vi "test TCX read (installed 71).vi"() -> ()   [LabVIEW 2011] (continued)
T14:01:31Z</Time><Position><LatitudeDegrees>35.863725</LatitudeDegrees><LongitudeDegrees>-78.910687</LongitudeDegrees></Position><AltitudeMeters>93.385</AltitudeMeters><DistanceMeters>7071.063</DistanceMeters><Cadence>74</Cadence><Extensions><TPX xmlns=\"http://www.garmin.com/xmlschemas/ActivityExtension/v2\"><Watts>109</Watts></TPX></Extensions></Trackpoint><Trackpoint><Time>2008-03-03T14:01:32Z</Time><Position><LatitudeDegrees>35.863710</LatitudeDegrees><LongitudeDegrees>-78.910596</LongitudeDegrees></Position><AltitudeMeters>93.385</AltitudeMeters><DistanceMeters>7079.492</DistanceMeters><Cadence>74</Cadence><Extensions><TPX xmlns=\"http://www.garmin.com/xmlschemas/ActivityExtension/v2\"><Watts>108</Watts></TPX></Extensions></Trackpoint><Trackpoint><Time>2008-03-03T14:01:33Z</Time><Position><LatitudeDegrees>35.863695</LatitudeDegrees><LongitudeDegrees>-78.910502</LongitudeDegrees></Position><AltitudeMeters>92.905</AltitudeMeters><DistanceMeters>7088.167</DistanceMeters><Cadence>70</Cadence><Extensions><TPX xmlns=\"http://www.garmin.com/xmlschemas/ActivityExtension/v2\"><Watts>110</Watts></TPX></Extensions></Trackpoint><Trackpoint><Time>2008-03-03T14:01:34Z</Time><Position><LatitudeDegrees>35.863685</LatitudeDegrees><LongitudeDegrees>-78.910407</LongitudeDegrees></Position><AltitudeMeters>92.905</AltitudeMeters><DistanceMeters>7096.799</DistanceMeters><Cadence>71</Cadence><Extensions><TPX xmlns=\"http://www.garmin.com/xmlschemas/ActivityExtension/v2\"><Watts>119</Watts></TPX></Extensions></Trackpoint><Trackpoint><Time>2008-03-03T14:01:35Z</Time><Position><LatitudeDegrees>35.863670</LatitudeDegrees><LongitudeDegrees>-78.910309</LongitudeDegrees></Position><AltitudeMeters>92.424</AltitudeMeters><DistanceMeters>7105.804</DistanceMeters><Cadence>74</Cadence><Extensions><TPX xmlns=\"http://www.garmin.com/xmlschemas/ActivityExtension/v2\"><Watts>107</Watts></TPX></Extensions></Trackpoint><Trackpoint><Time>2008-03-03T14:01:36Z</Time><Position><LatitudeDegrees>35.863654</LatitudeDegrees><LongitudeDegrees>-78.910210</LongitudeDegrees></Position><AltitudeMeters>92.424</AltitudeMeters><DistanceMeters>7114.917</DistanceMeters><Cadence>75</Cadence><Extensions><TPX xmlns=\"http://www.garmin.com/xmlschemas/ActivityExtension/v2\"><Watts>96</Watts></TPX></Extensions></Trackpoint><Trackpoint><Time>2008-03-03T14:01:37Z</Time><Position><LatitudeDegrees>35.863638</LatitudeDegrees><LongitudeDegrees>-78.910109</LongitudeDegrees></Position><AltitudeMeters>91.463</AltitudeMeters><DistanceMeters>7124.211</DistanceMeters><Cadence>76</Cadence><Extensions><TPX xmlns=\"http://www.garmin.com/xmlschemas/ActivityExtension/v2\"><Watts>95</Watts></TPX></Extensions></Trackpoint><Trackpoint><Time>2008-03-03T14:01:38Z</Time><Position><LatitudeDegrees>35.863622</LatitudeDegrees><LongitudeDegrees>-78.910006</LongitudeDegrees></Position><AltitudeMeters>91.463</AltitudeMeters><DistanceMeters>7133.708</DistanceMeters><Cadence>77</Cadence><Extensions><TPX xmlns=\"http://www.garmin.com/xmlschemas/ActivityExtension/v2\"><Watts>98</Watts></TPX></Extensions></Trackpoint><Trackpoint><Time>2008-03-03T14:01:39Z</Time><Position><LatitudeDegrees>35.863607</LatitudeDegrees><LongitudeDegrees>-78.909902</LongitudeDegrees></Position><AltitudeMeters>90.982</AltitudeMeters><DistanceMeters>7143.275</DistanceMeters><Cadence>77</Cadence><Extensions><TPX xmlns=\"http://www.garmin.com/xmlschemas/ActivityExtension/v2\"><Watts>98</Watts></TPX></Extensions></Trackpoint><Trackpoint><Time>2008-03-03T14:01:40Z</Time><Position><LatitudeDegrees>35.863592</LatitudeDegrees><LongitudeDegrees>-78.909796</LongitudeDegrees></Position><AltitudeMeters>90.982</AltitudeMeters><DistanceMeters>7152.969</DistanceMeters><Cadence>79</Cadence><Extensions><TPX xmlns=\"http://www.garmin.com/xmlschemas/ActivityExtension/v2\"><Watts>114</Watts></TPX></Extensions></Trackpoint><Trackpoint><Time>2008-03-03T14:01:41Z</Time><Position><LatitudeDegrees>35.863576</LatitudeDegrees><LongitudeDegrees>-78.909689</LongitudeDegrees></Position><AltitudeMeters>90.982</AltitudeMeters><DistanceMeters>7162.816</DistanceMeters><Cadence>80</Cadence><Extensions><TPX xmlns=\"http://www.garmin.com/xmlschemas/ActivityExtension/v2\"><Watts>119</Watts></TPX></Extensions></Trackpoint><Trackpoint><Time>2008-03-03T14:01:42Z</Time><Position><LatitudeDegrees>35.863561</LatitudeDegrees><LongitudeDegrees>-78.909581</LongitudeDegrees></Position><AltitudeMeters>90.982</AltitudeMeters><DistanceMeters>7172.724</DistanceMeters><Cadence>81</Cadence><Extensions><TPX xmlns=\"http://www.garmin.com/xmlschemas/ActivityExtension/v2\"><Watts>127</Watts></TPX></Extensions></Trackpoint><Trackpoint><Time>2008-03-03T14:01:43Z</Time><Position><LatitudeDegrees>35.863542</LatitudeDegrees><LongitudeDegrees>-78.909472</LongitudeDegrees></Position><AltitudeMeters>90.501</AltitudeMeters><DistanceMeters>7182.813</DistanceMeters><Cadence>82</Cadence><Extensions><TPX xmlns=\"http://www.garmin.com/xmlschemas/ActivityExtension/v2\"><Watts>113</Watts></TPX></Extensions></Trackpoint><Trackpoint><Time>2008-03-03T14:01:44Z</Time><Position><LatitudeDegrees>35.863526</LatitudeDegrees><LongitudeDegrees>-78.909363</LongitudeDegrees></Position><AltitudeMeters>90.021</AltitudeMeters><DistanceMeters>7192.831</DistanceMeters><Cadence>82</Cadence><Extensions><TPX xmlns=\"http://www.garmin.com/xmlschemas/ActivityExtension/v2\"><Watts>120</Watts></TPX></Extensions></Trackpoint><Trackpoint><Time>2008-03-03T14:01:45Z</Time><Position><LatitudeDegrees>35.863510</LatitudeDegrees><LongitudeDegrees>-78.909253</LongitudeDegrees></Position><AltitudeMeters>89.540</AltitudeMeters><DistanceMeters>7202.898</DistanceMeters><Cadence>82</Cadence><Extensions><TPX xmlns=\"http://www.garmin.com/xmlschemas/ActivityExtension/v2\"><Watts>110</Watts></TPX></Extensions></Trackpoint><Trackpoint><Time>2008-03-03T14:01:46Z</Time><Position><LatitudeDegrees>35.863491</LatitudeDegrees><LongitudeDegrees>-78.909143</LongitudeDegrees></Position><AltitudeMeters>89.540</AltitudeMeters><DistanceMeters>7213.067</DistanceMeters><Cadence>83</Cadence><Extensions><TPX xmlns=\"http://www.garmin.com/xmlschemas/ActivityExtension/v2\"><Watts>105</Watts></TPX></Extensions></Trackpoint><Trackpoint><Time>2008-03-03T14:01:47Z</Time><Position><LatitudeDegrees>35.863470</LatitudeDegrees><LongitudeDegrees>-78.909031</LongitudeDegrees></Position><AltitudeMeters>89.540</AltitudeMeters><DistanceMeters>7223.420</DistanceMeters><Cadence>83</Cadence><Extensions><TPX xmlns=\"http://www.garmin.com/xmlschemas/ActivityExtension/v2\"><Watts>109</Watts></TPX></Extensions></Trackpoint><Trackpoint><Time>2008-03-03T14:01:48Z</Time><Position><LatitudeDegrees>35.863450</LatitudeDegrees><LongitudeDegrees>-78.908921</LongitudeDegrees></Position><AltitudeMeters>89.059</AltitudeMeters><DistanceMeters>7233.568</DistanceMeters><Cadence>83</Cadence><Extensions><TPX xmlns=\"http://www.garmin.com/xmlschemas/ActivityExtension/v2\"><Watts>110</Watts></TPX></Extensions></Trackpoint><Trackpoint><Time>2008-03-03T14:01:49Z</Time><Position><LatitudeDegrees>35.863429</LatitudeDegrees><LongitudeDegrees>-78.908812</LongitudeDegrees></Position><AltitudeMeters>89.059</AltitudeMeters><DistanceMeters>7243.720</DistanceMeters><Cadence>83</Cadence><Extensions><TPX xmlns=\"http://www.garmin.com/xmlschemas/ActivityExtension/v2\"><Watts>111</Watts></TPX></Extensions></Trackpoint><Trackpoint><Time>2008-03-03T14:01:50Z</Time><Position><LatitudeDegrees>35.863409</LatitudeDegrees><LongitudeDegrees>-78.908702</LongitudeDegrees></Position><AltitudeMeters>89.059</AltitudeMeters><DistanceMeters>7253.881</DistanceMeters><Cadence>82</Cadence><Extensions><TPX xmlns=\"http://www.garmin.com/xmlschemas/ActivityExtension/v2\"><Watts>118</Watts></TPX></Extensions></Trackpoint><Trackpoint><Time>2008-03-03T14:01:51Z</Time><Position><LatitudeDegrees>35.863386</LatitudeDegrees><LongitudeDegrees>-78.908594</LongitudeDegrees></Position><AltitudeMeters>89.540</AltitudeMeters><DistanceMeters>7263.956</DistanceMeters><Cadence>82</Cadence><Extensions><TPX xmlns=\"http://www.garmin.com/xmlschemas/ActivityExtension/v2\"><Watts>118</Watts></TPX></Extensions></Trackpoint><Trackpoint><Time>2008-03-03T14:01:52Z</Time><Position><LatitudeDegrees>35.863365</LatitudeDegrees><LongitudeDegrees>-78.908487</LongitudeDegrees></Position><AltitudeMeters>89.059</AltitudeMeters><DistanceMeters>7273.903</DistanceMeters><Cadence>80</Cadence><Extensions><TPX xmlns=\"http://www.garmin.com/xmlschemas/ActivityExtension/v2\"><Watts>119</Watts></TPX></Extensions></Trackpoint><Trackpoint><Time>2008-03-03T14:01:53Z</Time><Position><LatitudeDegrees>35.863341</LatitudeDegrees><LongitudeDegrees>-78.908381</LongitudeDegrees></Position><AltitudeMeters>89.059</AltitudeMeters><DistanceMeters>7283.836</DistanceMeters><Cadence>80</Cadence><Extensions><TPX xmlns=\"http://www.garmin.com/xmlschemas/ActivityExtension/v2\"><Watts>124</Watts></TPX></Extensions></Trackpoint><Trackpoint><Time>2008-03-03T14:01:54Z</Time><Position><LatitudeDegrees>35.863310</LatitudeDegrees><LongitudeDegrees>-78.908278</LongitudeDegrees></Position><AltitudeMeters>89.059</AltitudeMeters><DistanceMeters>7293.733</DistanceMeters><Cadence>80</Cadence><Extensions><TPX xmlns=\"http://www.garmin.com/xmlschemas/ActivityExtension/v2\"><Watts>127</Watts></TPX></Extensions></Trackpoint><Trackpoint><Time>2008-03-03T14:01:55Z</Time><Position><LatitudeDegrees>35.863282</LatitudeDegrees><LongitudeDegrees>-78.908177</LongitudeDegrees></Position><AltitudeMeters>88.579</AltitudeMeters><DistanceMeters>7303.308</DistanceMeters><Cadence>77</Cadence><Extensions><TPX xmlns=\"http://www.garmin.com/xmlschemas/ActivityExtension/v2\"><Watts>143</Watts></TPX></Extensions></Trackpoint><Trackpoint><Time>2008-03-03T14:01:56Z</Time><Position><LatitudeDegrees>35.863254</LatitudeDegrees><LongitudeDegrees>-78.908080</LongitudeDegrees></Position><AltitudeMeters>89.059</AltitudeMeters><DistanceMeters>7312.629</DistanceMeters><Cadence>76</Cadence><Extensions><TPX xmlns=\"http://www.garmin.com/xmlschemas/ActivityExtension/v2\"><Watts>158</Watts></TPX></Extensions></Trackpoint><Trackpoint><Time>2008-03-03T14:01:57Z</Time><Position><LatitudeDegrees>35.863228</LatitudeDegrees><LongitudeDegrees>-78.907986</LongitudeDegrees></Position><AltitudeMeters>89.540</AltitudeMeters><DistanceMeters>7321.532</DistanceMeters><Cadence>73</Cadence><Extensions><TPX xmlns=\"http://www.garmin.com/xmlschemas/ActivityExtension/v2\"><Watts>164</Watts></TPX></Extensions></Trackpoint><Trackpoint><Time>2008-03-03T14:01:58Z</Time><Position><LatitudeDegrees>35.863199</LatitudeDegrees><LongitudeDegrees>-78.907895</LongitudeDegrees></Position><AltitudeMeters>89.540</AltitudeMeters><DistanceMeters>7330.394</DistanceMeters><Cadence>70</Cadence><Extensions><TPX xmlns=\"http://www.garmin.com/xmlschemas/ActivityExtension/v2\"><Watts>168</Watts></TPX></Extensions></Trackpoint><Trackpoint><Time>2008-03-03T14:01:59Z</Time><Position><LatitudeDegrees>35.863176</LatitudeDegrees><LongitudeDegrees>-78.907807</LongitudeDegrees></Position><AltitudeMeters>89.540</AltitudeMeters><DistanceMeters>7338.662</DistanceMeters><Cadence>70</Cadence><Extensions><TPX xmlns=\"http://www.garmin.com/xmlschemas/ActivityExtension/v2\"><Watts>170</Watts></TPX></Extensions></Trackpoint><Trackpoint><Time>2008-03-03T14:02:00Z</Time><Position><LatitudeDegrees>35.863156</LatitudeDegrees><LongitudeDegrees>-78.907723</LongitudeDegrees></Position><AltitudeMeters>89.540</AltitudeMeters><DistanceMeters>7346.539</DistanceMeters><Cadence>76</Cadence><Extensions><TPX xmlns=\"http://www.garmin.com/xmlschemas/ActivityExtension/v2\"><Watts>163</Watts></TPX></Extensions></Trackpoint><Trackpoint><Time>2008-03-03T14:02:01Z</Time><Position><LatitudeDegrees>35.863135</LatitudeDegrees><LongitudeDegrees>-78.907643</LongitudeDegrees></Position><AltitudeMeters>89.540</AltitudeMeters><DistanceMeters>7354.126</DistanceMeters><Cadence>80</Cadence><Extensions><TPX xmlns=\"http://www.garmin.com/xmlschemas/ActivityExtension/v2\"><Watts>164</Watts></TPX></Extensions></Trackpoint><Trackpoint><Time>2008-03-03T14:02:02Z</Time><Position><LatitudeDegrees>35.863115</LatitudeDegrees><LongitudeDegrees>-78.907565</LongitudeDegrees></Position><AltitudeMeters>90.501</AltitudeMeters><DistanceMeters>7361.460</DistanceMeters><Cadence>77</Cadence><Extensions><TPX xmlns=\"http://www.garmin.com/xmlschemas/ActivityExtension/v2\"><Watts>190</Watts></TPX></Extensions></Trackpoint><Trackpoint><Time>2008-03-03T14:02:03Z</Time><Position><LatitudeDegrees>35.863091</LatitudeDegrees><LongitudeDegrees>-78.907489</LongitudeDegrees></Position><AltitudeMeters>90.501</AltitudeMeters><DistanceMeters>7368.861</DistanceMeters><Cadence>76</Cadence><Extensions><TPX xmlns=\"http://www.garmin.com/xmlschemas/ActivityExtension/v2\"><Watts>233</Watts></TPX></Extensions></Trackpoint><Trackpoint><Time>2008-03-03T14:02:04Z</Time><Position><LatitudeDegrees>35.863071</LatitudeDegrees><LongitudeDegrees>-78.907413</LongitudeDegrees></Position><AltitudeMeters>90.501</AltitudeMeters><DistanceMeters>7376.071</DistanceMeters><Cadence>76</Cadence><Extensions><TPX xmlns=\"http://www.garmin.com/xmlschemas/ActivityExtension/v2\"><Watts>311</Watts></TPX></Extensions></Trackpoint><Trackpoint><Time>2008-03-03T14:02:05Z</Time><Position><LatitudeDegrees>35.863051</LatitudeDegrees><LongitudeDegrees>-78.907336</LongitudeDegrees></Position><AltitudeMeters>90.982</AltitudeMeters><DistanceMeters>7383.323</DistanceMeters><Cadence>76</Cadence><Extensions><TPX xmlns=\"http://www.garmin.com/xmlschemas/ActivityExtension/v2\"><Watts>376</Watts></TPX></Extensions></Trackpoint><Trackpoint><Time>2008-03-03T14:02:06Z</Time><Position><LatitudeDegrees>35.863031</LatitudeDegrees><LongitudeDegrees>-78.907260</LongitudeDegrees></Position><AltitudeMeters>91.463</AltitudeMeters><DistanceMeters>7390.527</DistanceMeters><Cadence>75</Cadence><Extensions><TPX xmlns=\"http://www.garmin.com/xmlschemas/ActivityExtension/v2\"><Watts>375</Watts></TPX></Extensions></Trackpoint><Trackpoint><Time>2008-03-03T14:02:07Z</Time><Position><LatitudeDegrees>35.863008</LatitudeDegrees><LongitudeDegrees>-78.907185</LongitudeDegrees></Position><AltitudeMeters>91.463</AltitudeMeters><DistanceMeters>7397.769</DistanceMeters><Cadence>75</Cadence><Extensions><TPX xmlns=\"http://www.garmin.com/xmlschemas/ActivityExtension/v2\"><Watts>366</Watts></TPX></Extensions></Trackpoint><Trackpoint><Time>2008-03-03T14:02:08Z</Time><Position><LatitudeDegrees>35.862984</LatitudeDegrees><LongitudeDegrees>-78.907112</LongitudeDegrees></Position><AltitudeMeters>91.943</AltitudeMeters><DistanceMeters>7404.936</DistanceMeters><Cadence>73</Cadence><Extensions><TPX xmlns=\"http://www.garmin.com/xmlschemas/ActivityExtension/v2\"><Watts>326</Watts></TPX></Extensions></Trackpoint><Trackpoint><Time>2008-03-03T14:02:09Z</Time><Position><LatitudeDegrees>35.862961</LatitudeDegrees><LongitudeDegrees>-78.907039</LongitudeDegrees></Position><AltitudeMeters>91.943</AltitudeMeters><DistanceMeters>7411.968</DistanceMeters><Cadence>73</Cadence><Extensions><TPX xmlns=\"http://www.garmin.com/xmlschemas/ActivityExtension/v2\"><Watts>326</Watts></TPX></Extensions></Trackpoint><Trackpoint><Time>2008-03-03T14:02:10Z</Time><Position><LatitudeDegrees>35.862937</LatitudeDegrees><LongitudeDegrees>-78.906968</LongitudeDegrees></Position><AltitudeMeters>91.943</AltitudeMeters><DistanceMeters>7418.891</DistanceMeters><Cadence>72</Cadence><Extensions><TPX xmlns=\"http://www.garmin.com/xmlschemas/ActivityExtension/v2\"><Watts>311</Watts></TPX></Extensions></Trackpoint><Trackpoint><Time>2008-03-03T14:02:11Z</Time><Position><LatitudeDegrees>35.862914</LatitudeDegrees><LongitudeDegrees>-78.906899</LongitudeDegrees></Position><AltitudeMeters>92.424</AltitudeMeters><DistanceMeters>7425.608</DistanceMeters><Cadence>70</Cadence><Extensions><TPX xmlns=\"http://www.garmin.com/xmlschemas/ActivityExtension/v2\"><Watts>296</Watts></TPX></Extensions></Trackpoint><Trackpoint><Time>2008-03-03T14:02:12Z</Time><Position><LatitudeDegrees>35.862890</LatitudeDegrees><LongitudeDegrees>-78.906832</LongitudeDegrees></Position><AltitudeMeters>92.424</AltitudeMeters><DistanceMeters>7432.226</DistanceMeters><Cadence>70</Cadence><Extensions><TPX xmlns=\"http://www.garmin.com/xmlschemas/ActivityExtension/v2\"><Watts>283</Watts></TPX></Extensions></Trackpoint><Trackpoint><Time>2008-03-03T14:02:13Z</Time><Position><LatitudeDegrees>35.862866</LatitudeDegrees><LongitudeDegrees>-78.906766</LongitudeDegrees></Position><AltitudeMeters>92.905</AltitudeMeters><DistanceMeters>7438.779</DistanceMeters><Cadence>69</Cadence><Extensions><TPX xmlns=\"http://www.garmin.com/xmlschemas/ActivityExtension/v2\"><Watts>271</Watts></TPX></Extensions></Trackpoint><Trackpoint><Time>2008-03-03T14:02:14Z</Time><Position><LatitudeDegrees>35.862841</LatitudeDegrees><LongitudeDegrees>-78.906700</LongitudeDegrees></Position><AltitudeMeters>92.905</AltitudeMeters><DistanceMeters>7445.341</DistanceMeters><Cadence>68</Cadence><Extensions><TPX xmlns=\"http://www.garmin.com/xmlschemas/ActivityExtension/v2\"><Watts>265</Watts></TPX></Extensions></Trackpoint><Trackpoint><Time>2008-03-03T14:02:15Z</Time><Position><LatitudeDegrees>35.862814</LatitudeDegrees><LongitudeDegrees>-78.906635</LongitudeDegrees></Position><AltitudeMeters>92.905</AltitudeMeters><DistanceMeters>7451.964</DistanceMeters><Cadence>69</Cadence><Extensions><TPX xmlns=\"http://www.garmin.com/xmlschemas/ActivityExtension/v2\"><Watts>259</Watts></TPX></Extensions></Trackpoint><Trackpoint><Time>2008-03-03T14:02:16Z</Time><Position><LatitudeDegrees>35.862788</LatitudeDegrees><LongitudeDegrees>-78.906569</LongitudeDegrees></Position><AltitudeMeters>92.905</AltitudeMeters><DistanceMeters>7458.573</DistanceMeters><Cadence>69</Cadence><Extensions><TPX xmlns=\"http://www.garmin.com/xmlschemas/ActivityExtension/v2\"><Watts>224</Watts></TPX></Extensions></Trackpoint><Trackpoint><Time>2008-03-03T14:02:17Z</Time><Position><LatitudeDegrees>35.862762</LatitudeDegrees><LongitudeDegrees>-78.906502</LongitudeDegrees></Position><AltitudeMeters>93.385</AltitudeMeters><DistanceMeters>7465.271</DistanceMeters><Cadence>70</Cadence><Extensions><TPX xmlns=\"http://www.garmin.com/xmlschemas/ActivityExtension/v2\"><Watts>183</Watts></TPX></Extensions></Trackpoint><Trackpoint><Time>2008-03-03T14:02:18Z</Time><Position><LatitudeDegrees>35.862733</LatitudeDegrees><LongitudeDegrees>-78.906434</LongitudeDegrees></Position><AltitudeMeters>93.385</AltitudeMeters><DistanceMeters>7472.209</DistanceMeters><Cadence>71</Cadence><Extensions><TPX xmlns=\"http://www.garmin.com/xmlschemas/ActivityExtension/v2\"><Watts>175</Watts></TPX></Extensions></Trackpoint><Trackpoint><Time>2008-03-03T14:02:19Z</Time><Position><LatitudeDegrees>35.862707</LatitudeDegrees><LongitudeDegrees>-78.906364</LongitudeDegrees></Position><AltitudeMeters>93.385</AltitudeMeters><DistanceMeters>7479.178</DistanceMeters><Cadence>74</Cadence><Extensions><TPX xmlns=\"http://www.garmin.com/xmlschemas/ActivityExtension/v2\"><Watts>127</Watts></TPX></Extensions></Trackpoint><Trackpoint><Time>2008-03-03T14:02:20Z</Time><Position><LatitudeDegrees>35.862678</LatitudeDegrees><LongitudeDegrees>-78.906293</LongitudeDegrees></Position><AltitudeMeters>93.385</AltitudeMeters><DistanceMeters>7486.349</DistanceMeters><Cadence>76</Cadence><Extensions><TPX xmlns=\"http://www.garmin.com/xmlschemas/ActivityExtension/v2\"><Watts>106</Watts></TPX></Extensions></Trackpoint><Trackpoint><Time>2008-03-03T14:02:21Z</Time><Position><LatitudeDegrees>35.862649</LatitudeDegrees><LongitudeDegrees>-78.906220</LongitudeDegrees></Position><AltitudeMeters>92.905</AltitudeMeters><DistanceMeters>7493.638</DistanceMeters><Cadence>76</Cadence><Extensions><TPX xmlns=\"http://www.garmin.com/xmlschemas/ActivityExtension/v2\"><Watts>105</Watts></TPX></Extensions></Trackpoint><Trackpoint><Time>2008-03-03T14:02:22Z</Time><Position><LatitudeDegrees>35.862616</LatitudeDegrees><LongitudeDegrees>-78.906145</LongitudeDegrees></Position><AltitudeMeters>92.905</AltitudeMeters><DistanceMeters>7501.450</DistanceMeters><Cadence>74</Cadence><Extensions><TPX xmlns=\"http://www.garmin.com/xmlschemas/ActivityExtension/v2\"><Watts>105</Watts></TPX></Extensions></Trackpoint><Trackpoint><Time>2008-03-03T14:02:23Z</Time><Position><LatitudeDegrees>35.862577</LatitudeDegrees><LongitudeDegrees>-78.906066</LongitudeDegrees></Position><AltitudeMeters>92.905</AltitudeMeters><DistanceMeters>7509.722</DistanceMeters><Cadence>74</Cadence><Extensions><TPX xmlns=\"http://www.garmin.com/xmlschemas/ActivityExtension/v2\"><Watts>107</Watts></TPX></Extensions></Trackpoint><Trackpoint><Time>2008-03-03T14:02:24Z</Time><Position><LatitudeDegrees>35.862538</LatitudeDegrees><LongitudeDegrees>-78.905985</LongitudeDegrees></Position><AltitudeMeters>92.424</AltitudeMeters><DistanceMeters>7518.321</DistanceMeters><Cadence>79</Cadence><Extensions><TPX xmlns=\"http://www.garmin.com/xmlschemas/ActivityExtension/v2\"><Watts>149</Watts></TPX></Extensions></Trackpoint><Trackpoint><Time>2008-03-03T14:02:25Z</Time><Position><LatitudeDegrees>35.862503</LatitudeDegrees><LongitudeDegrees>-78.905901</LongitudeDegrees></Position><AltitudeMeters>92.424</AltitudeMeters><DistanceMeters>7526.838</DistanceMeters><Cadence>81</Cadence><Extensions><TPX xmlns=\"http://www.garmin.com/xmlschemas/ActivityExtension/v2\"><Watts>149</Watts></TPX></Extensions></Trackpoint><Trackpoint><Time>2008-03-03T14:02:26Z</Time><Position><LatitudeDegrees>35.862465</LatitudeDegrees><LongitudeDegrees>-78.905813</LongitudeDegrees></Position><AltitudeMeters>91.943</AltitudeMeters><DistanceMeters>7535.852</DistanceMeters><Cadence>84</Cadence><Extensions><TPX xmlns=\"http://www.garmin.com/xmlschemas/ActivityExtension/v2\"><Watts>152</Watts></TPX></Extensions></Trackpoint><Trackpoint><Time>2008-03-03T14:02:27Z</Time><Position><LatitudeDegrees>35.862426</LatitudeDegrees><LongitudeDegrees>-78.905724</LongitudeDegrees></Position><AltitudeMeters>91.463</AltitudeMeters><DistanceMeters>7544.979</DistanceMeters><Cadence>86</Cadence><Extensions><TPX xmlns=\"http://www.garmin.com/xmlschemas/ActivityExtension/v2\"><Watts>137</Watts></TPX></Extensions></Trackpoint><Trackpoint><Time>2008-03-03T14:02:28Z</Time><Position><LatitudeDegrees>35.862387</LatitudeDegrees><LongitudeDegrees>-78.905633</LongitudeDegrees></Position><AltitudeMeters>92.424</AltitudeMeters><DistanceMeters>7554.277</DistanceMeters><Cadence>86</Cadence><Extensions><TPX xmlns=\"http://www.garmin.com/xmlschemas/ActivityExtension/v2\"><Watts>137</Watts></TPX></Extensions></Trackpoint><Trackpoint><Time>2008-03-03T14:02:29Z</Time><Position><LatitudeDegrees>35.862347</LatitudeDegrees><LongitudeDegrees>-78.905540</LongitudeDegrees></Position><AltitudeMeters>91.463</AltitudeMeters><DistanceMeters>7563.752</DistanceMeters><Cadence>88</Cadence><Extensions><TPX xmlns=\"http://www.garmin.com/xmlschemas/ActivityExtension/v2\"><Watts>137</Watts></TPX></Extensions></Trackpoint><Trackpoint><Time>2008-03-03T14:02:30Z</Time><Position><LatitudeDegrees>35.862308</LatitudeDegrees><LongitudeDegrees>-78.905447</LongitudeDegrees></Position><AltitudeMeters>91.463</AltitudeMeters><DistanceMeters>7573.245</DistanceMeters><Cadence>87</Cadence><Extensions><TPX xmlns=\"http://www.garmin.com/xmlschemas/ActivityExtension/v2\"><Watts>150</Watts></TPX></Extensions></Trackpoint><Trackpoint><Time>2008-03-03T14:02:31Z</Time><Position><LatitudeDegrees>35.862269</LatitudeDegrees><LongitudeDegrees>-78.905354</LongitudeDegrees></Position><AltitudeMeters>91.463</AltitudeMeters><DistanceMeters>7582.627</DistanceMeters><Cadence>87</Cadence><Extensions><TPX xmlns=\"http://www.garmin.com/xmlschemas/ActivityExtension/v2\"><Watts>149</Watts></TPX></Extensions></Trackpoint><Trackpoint><Time>2008-03-03T14:02:32Z</Time><Position><LatitudeDegrees>35.862232</LatitudeDegrees><LongitudeDegrees>-78.905262</LongitudeDegrees></Position><AltitudeMeters>91.463</AltitudeMeters><DistanceMeters>7591.958</DistanceMeters><Cadence>86</Cadence><Extensions><TPX xmlns=\"http://www.garmin.com/xmlschemas/ActivityExtension/v2\"><Watts>167</Watts></TPX></Extensions></Trackpoint><Trackpoint><Time>2008-03-03T14:02:33Z</Time><Position><LatitudeDegrees>35.862199</LatitudeDegrees><LongitudeDegrees>-78.905168</LongitudeDegrees></Position><AltitudeMeters>91.463</AltitudeMeters><DistanceMeters>7601.143</DistanceMeters><Cadence>86</Cadence><Extensions><TPX xmlns=\"http://www.garmin.com/xmlschemas/ActivityExtension/v2\"><Watts>166</Watts></TPX></Extensions></Trackpoint><Trackpoint><Time>2008-03-03T14:02:34Z</Time><Position><LatitudeDegrees>35.862167</LatitudeDegrees><LongitudeDegrees>-78.905075</LongitudeDegrees></Position><AltitudeMeters>91.463</AltitudeMeters><DistanceMeters>7610.301</DistanceMeters><Cadence>85</Cadence><Extensions><TPX xmlns=\"http://www.garmin.com/xmlschemas/ActivityExtension/v2\"><Watts>166</Watts></TPX></Extensions></Trackpoint><Trackpoint><Time>2008-03-03T14:02:35Z</Time><Position><LatitudeDegrees>35.862140</LatitudeDegrees><LongitudeDegrees>-78.904980</LongitudeDegrees></Position><AltitudeMeters>91.463</AltitudeMeters><DistanceMeters>7619.282</DistanceMeters><Cadence>83</Cadence><Extensions><TPX xmlns=\"http://www.garmin.com/xmlschemas/ActivityExtension/v2\"><Watts>162</Watts></TPX></Extensions></Trackpoint><Trackpoint><Time>2008-03-03T14:02:36Z</Time><Position><LatitudeDegrees>35.862123</LatitudeDegrees><LongitudeDegrees>-78.904885</LongitudeDegrees></Position><AltitudeMeters>91.463</AltitudeMeters><DistanceMeters>7628.092</DistanceMeters><Cadence>81</Cadence><Extensions><TPX xmlns=\"http://www.garmin.com/xmlschemas/ActivityExtension/v2\"><Watts>154</Watts></TPX></Extensions></Trackpoint><Trackpoint><Time>2008-03-03T14:02:37Z</Time><Position><LatitudeDegrees>35.862111</LatitudeDegrees><LongitudeDegrees>-78.904789</LongitudeDegrees></Position><AltitudeMeters>91.943</AltitudeMeters><DistanceMeters>7636.858</DistanceMeters><Cadence>81</Cadence><Extensions><TPX xmlns=\"http://www.garmin.com/xmlschemas/ActivityExtension/v2\"><Watts>149</Watts></TPX></Extensions></Trackpoint><Trackpoint><Time>2008-03-03T14:02:38Z</Time><Position><LatitudeDegrees>35.862110</LatitudeDegrees><LongitudeDegrees>-78.904692</LongitudeDegrees></Position><AltitudeMeters>91.463</AltitudeMeters><DistanceMeters>7645.604</DistanceMeters><Cadence>81</Cadence><Extensions><TPX xmlns=\"http://www.garmin.com/xmlschemas/ActivityExtension/v2\"><Watts>143</Watts></TPX></Extensions></Trackpoint><Trackpoint><Time>2008-03-03T14:02:39Z</Time><Position><LatitudeDegrees>35.862115</LatitudeDegrees><LongitudeDegrees>-78.904595</LongitudeDegrees></Position><AltitudeMeters>91.463</AltitudeMeters><DistanceMeters>7654.416</DistanceMeters><Cadence>82</Cadence><Extensions><TPX xmlns=\"http://www.garmin.com/xmlschemas/ActivityExtension/v2\"><Watts>129</Watts></TPX></Extensions></Trackpoint><Trackpoint><Time>2008-03-03T14:02:40Z</Time><Position><LatitudeDegrees>35.862128</LatitudeDegrees><LongitudeDegrees>-78.904496</LongitudeDegrees></Position><AltitudeMeters>90.982</AltitudeMeters><DistanceMeters>7663.441</DistanceMeters><Cadence>82</Cadence><Extensions><TPX xmlns=\"http://www.garmin.com/xmlschemas/ActivityExtension/v2\"><Watts>129</Watts></TPX></Extensions></Trackpoint><Trackpoint><Time>2008-03-03T14:02:41Z</Time><Position><LatitudeDegrees>35.862146</LatitudeDegrees><LongitudeDegrees>-78.904397</LongitudeDegrees></Position><AltitudeMeters>90.982</AltitudeMeters><DistanceMeters>7672.676</DistanceMeters><Cadence>85</Cadence><Extensions><TPX xmlns=\"http://www.garmin.com/xmlschemas/ActivityExtension/v2\"><Watts>119</Watts></TPX></Extensions></Trackpoint><Trackpoint><Time>2008-03-03T14:02:42Z</Time><Position><LatitudeDegrees>35.862170</LatitudeDegrees><LongitudeDegrees>-78.904297</LongitudeDegrees></Position><AltitudeMeters>90.982</AltitudeMeters><DistanceMeters>7682.102</DistanceMeters><Cadence>86</Cadence><Extensions><TPX xmlns=\"http://www.garmin.com/xmlschemas/ActivityExtension/v2\"><Watts>117</Watts></TPX></Extensions></Trackpoint><Trackpoint><Time>2008-03-03T14:02:43Z</Time><Position><LatitudeDegrees>35.862199</LatitudeDegrees><LongitudeDegrees>-78.904198</LongitudeDegrees></Position><AltitudeMeters>90.982</AltitudeMeters><DistanceMeters>7691.604</DistanceMeters><Cadence>86</Cadence><Extensions><TPX xmlns=\"http://www.garmin.com/xmlschemas/ActivityExtension/v2\"><Watts>107</Watts></TPX></Extensions></Trackpoint><Trackpoint><Time>2008-03-03T14:02:44Z</Time><Position><LatitudeDegrees>35.862231</LatitudeDegrees><LongitudeDegrees>-78.904100</LongitudeDegrees></Position><AltitudeMeters>90.501</AltitudeMeters><DistanceMeters>7701.092</DistanceMeters><Cadence>87</Cadence><Extensions><TPX xmlns=\"http://www.garmin.com/xmlschemas/ActivityExtension/v2\"><Watts>115</Watts></TPX></Extensions></Trackpoint><Trackpoint><Time>2008-03-03T14:02:45Z</Time><Position><LatitudeDegrees>35.862262</LatitudeDegrees><LongitudeDegrees>-78.904002</LongitudeDegrees></Position><AltitudeMeters>90.501</AltitudeMeters><DistanceMeters>7710.564</DistanceMeters><Cadence>87</Cadence><Extensions><TPX xmlns=\"http://www.garmin.com/xmlschemas/ActivityExtension/v2\"><Watts>113</Watts></TPX></Extensions></Trackpoint><Trackpoint><Time>2008-03-03T14:02:46Z</Time><Position><LatitudeDegrees>35.862294</LatitudeDegrees><LongitudeDegrees>-78.903905</LongitudeDegrees></Position><AltitudeMeters>90.982</AltitudeMeters><DistanceMeters>7720.042</DistanceMeters><Cadence>87</Cadence><Extensions><TPX xmlns=\"http://www.garmin.com/xmlschemas/ActivityExtension/v2\"><Watts>112</Watts></TPX></Extensions></Trackpoint><Trackpoint><Time>2008-03-03T14:02:47Z</Time><Position><LatitudeDegrees>35.862327</LatitudeDegrees><LongitudeDegrees>-78.903811</LongitudeDegrees></Position><AltitudeMeters>90.982</AltitudeMeters><DistanceMeters>7729.342</DistanceMeters><Cadence>85</Cadence><Extensions><TPX xmlns=\"http://www.garmin.com/xmlschemas/ActivityExtension/v2\"><Watts>114</Watts></TPX></Extensions></Trackpoint><Trackpoint><Time>2008-03-03T14:02:48Z</Time><Position><LatitudeDegrees>35.862359</LatitudeDegrees><LongitudeDegrees>-78.903717</LongitudeDegrees></Position><AltitudeMeters>90.501</AltitudeMeters><DistanceMeters>7738.435</DistanceMeters><Cadence>84</Cadence><Extensions><TPX xmlns=\"http://www.garmin.com/xmlschemas/ActivityExtension/v2\"><Watts>114</Watts></TPX></Extensions></Trackpoint><Trackpoint><Time>2008-03-03T14:02:49Z</Time><Position><LatitudeDegrees>35.862388</LatitudeDegrees><LongitudeDegrees>-78.903627</LongitudeDegrees></Position><AltitudeMeters>90.501</AltitudeMeters><DistanceMeters>7747.194</DistanceMeters><Cadence>79</Cadence><Extensions><TPX xmlns=\"http://www.garmin.com/xmlschemas/ActivityExtension/v2\"><Watts>121</Watts></TPX></Extensions></Trackpoint><Trackpoint><Time>2008-03-03T14:02:50Z</Time><Position><LatitudeDegrees>35.862417</LatitudeDegrees><LongitudeDegrees>-78.903541</LongitudeDegrees></Position><AltitudeMeters>90.501</AltitudeMeters><DistanceMeters>7755.565</DistanceMeters><Cadence>77</Cadence><Extensions><TPX xmlns=\"http://www.garmin.com/xmlschemas/ActivityExtension/v2\"><Watts>124</Watts></TPX></Extensions></Trackpoint><Trackpoint><Time>2008-03-03T14:02:51Z</Time><Position><LatitudeDegrees>35.862445</LatitudeDegrees><LongitudeDegrees>-78.903459</LongitudeDegrees></Position><AltitudeMeters>90.501</AltitudeMeters><DistanceMeters>7763.628</DistanceMeters><Cadence>71</Cadence><Extensions><TPX xmlns=\"http://www.garmin.com/xmlschemas/ActivityExtension/v2\"><Watts>146</Watts></TPX></Extensions></Trackpoint><Trackpoint><Time>2008-03-03T14:02:52Z</Time><Position><LatitudeDegrees>35.862470</LatitudeDegrees><LongitudeDegrees>-78.903380</LongitudeDegrees></Position><AltitudeMeters>90.501</AltitudeMeters><DistanceMeters>7771.172</DistanceMeters><Cadence>71</Cadence><Extensions><TPX xmlns=\"http://www.garmin.com/xmlschemas/ActivityExtension/v2\"><Watts>145</Watts></TPX></Extensions></Trackpoint><Trackpoint><Time>2008-03-03T14:02:53Z</Time><Position><LatitudeDegrees>35.862494</LatitudeDegrees><LongitudeDegrees>-78.903306</LongitudeDegrees></Position><AltitudeMeters>90.982</AltitudeMeters><DistanceMeters>7778.396</DistanceMeters><Cadence>73</Cadence><Extensions><TPX xmlns=\"http://www.garmin.com/xmlschemas/ActivityExtension/v2\"><Watts>148</Watts></TPX></Extensions></Trackpoint><Trackpoint><Time>2008-03-03T14:02:54Z</Time><Position><LatitudeDegrees>35.862517</LatitudeDegrees><LongitudeDegrees>-78.903234</LongitudeDegrees></Position><AltitudeMeters>90.982</AltitudeMeters><DistanceMeters>7785.336</DistanceMeters><Cadence>72</Cadence><Extensions><TPX xmlns=\"http://www.garmin.com/xmlschemas/ActivityExtension/v2\"><Watts>168</Watts></TPX></Extensions></Trackpoint><Trackpoint><Time>2008-03-03T14:02:55Z</Time><Position><LatitudeDegrees>35.862540</LatitudeDegrees><LongitudeDegrees>-78.903163</LongitudeDegrees></Position><AltitudeMeters>91.463</AltitudeMeters><DistanceMeters>7792.307</DistanceMeters><Cadence>72</Cadence><Extensions><TPX xmlns=\"http://www.garmin.com/xmlschemas/ActivityExtension/v2\"><Watts>259</Watts></TPX></Extensions></Trackpoint><Trackpoint><Time>2008-03-03T14:02:56Z</Time><Position><LatitudeDegrees>35.862562</LatitudeDegrees><LongitudeDegrees>-78.903092</LongitudeDegrees></Position><AltitudeMeters>91.943</AltitudeMeters><DistanceMeters>7799.153</DistanceMeters><Cadence>73</Cadence><Extensions><TPX xmlns=\"http://www.garmin.com/xmlschemas/ActivityExtension/v2\"><Watts>364</Watts></TPX></Extensions></Trackpoint><Trackpoint><Time>2008-03-03T14:02:57Z</Time><Position><LatitudeDegrees>35.862582</LatitudeDegrees><LongitudeDegrees>-78.903019</LongitudeDegrees></Position><AltitudeMeters>91.943</AltitudeMeters><DistanceMeters>7806.098</DistanceMeters><Cadence>75</Cadence><Extensions><TPX xmlns=\"http://www.garmin.com/xmlschemas/ActivityExtension/v2\"><Watts>417</Watts></TPX></Extensions></Trackpoint><Trackpoint><Time>2008-03-03T14:02:58Z</Time><Position><LatitudeDegrees>35.862604</LatitudeDegrees><LongitudeDegrees>-78.902945</LongitudeDegrees></Position><AltitudeMeters>91.943</AltitudeMeters><DistanceMeters>7813.264</DistanceMeters><Cadence>75</Cadence><Extensions><TPX xmlns=\"http://www.garmin.com/xmlschemas/ActivityExtension/v2\"><Watts>415</Watts></TPX></Extensions></Trackpoint><Trackpoint><Time>2008-03-03T14:02:59Z</Time><Position><LatitudeDegrees>35.862629</LatitudeDegrees><LongitudeDegrees>-78.902868</LongitudeDegrees></Position><AltitudeMeters>92.424</AltitudeMeters><DistanceMeters>7820.747</DistanceMeters><Cadence>78</Cadence><Extensions><TPX xmlns=\"http://www.garmin.com/xmlschemas/ActivityExtension/v2\"><Watts>438</Watts></TPX></Extensions></Trackpoint><Trackpoint><Time>2008-03-03T14:03:00Z</Time><Position><LatitudeDegrees>35.862656</LatitudeDegrees><LongitudeDegrees>-78.902789</LongitudeDegrees></Position><AltitudeMeters>92.424</AltitudeMeters><DistanceMeters>7828.511</DistanceMeters><Cadence>80</Cadence><Extensions><TPX xmlns=\"http://www.garmin.com/xmlschemas/ActivityExtension/v2\"><Watts>433</Watts></TPX></Extensions></Trackpoint><Trackpoint><Time>2008-03-03T14:03:01Z</Time><Position><LatitudeDegrees>35.862681</LatitudeDegrees><LongitudeDegrees>-78.902708</LongitudeDegrees></Position><AltitudeMeters>92.905</AltitudeMeters><DistanceMeters>7836.369</DistanceMeters><Cadence>82</Cadence><Extensions><TPX xmlns=\"http://www.garmin.com/xmlschemas/ActivityExtension/v2\"><Watts>432</Watts></TPX></Extensions></Trackpoint><Trackpoint><Time>2008-03-03T14:03:02Z</Time><Position><LatitudeDegrees>35.862707</LatitudeDegrees><LongitudeDegrees>-78.902625</LongitudeDegrees></Position><AltitudeMeters>92.905</AltitudeMeters><DistanceMeters>7844.309</DistanceMeters><Cadence>83</Cadence><Extensions><TPX xmlns=\"http://www.garmin.com/xmlschemas/ActivityExtension/v2\"><Watts>405</Watts></TPX></Extensions></Trackpoint><Trackpoint><Time>2008-03-03T14:03:03Z</Time><Position><LatitudeDegrees>35.862733</LatitudeDegrees><LongitudeDegrees>-78.902543</LongitudeDegrees></Position><AltitudeMeters>93.385</AltitudeMeters><DistanceMeters>7852.350</DistanceMeters><Cadence>83</Cadence><Extensions><TPX xmlns=\"http://www.garmin.com/xmlschemas/ActivityExtension/v2\"><Watts>357</Watts></TPX></Extensions></Trackpoint><Trackpoint><Time>2008-03-03T14:03:04Z</Time><Position><LatitudeDegrees>35.862758</LatitudeDegrees><LongitudeDegrees>-78.902459</LongitudeDegrees></Position><AltitudeMeters>93.385</AltitudeMeters><DistanceMeters>7860.332</DistanceMeters><Cadence>83</Cadence><Extensions><TPX xmlns=\"http://www.garmin.com/xmlschemas/ActivityExtension/v2\"><Watts>314</Watts></TPX></Extensions></Trackpoint><Trackpoint><Time>2008-03-03T14:03:05Z</Time><Position><LatitudeDegrees>35.862786</LatitudeDegrees><LongitudeDegrees>-78.902377</LongitudeDegrees></Position><AltitudeMeters>93.385</AltitudeMeters><DistanceMeters>7868.415</DistanceMeters><Cadence>83</Cadence><Extensions><TPX xmlns=\"http://www.garmin.com/xmlschemas/ActivityExtension/v2\"><Watts>271</Watts></TPX></Extensions></Trackpoint><Trackpoint><Time>2008-03-03T14:03:06Z</Time><Position><LatitudeDegrees>35.862811</LatitudeDegrees><LongitudeDegrees>-78.902295</LongitudeDegrees></Position><AltitudeMeters>93.385</AltitudeMeters><DistanceMeters>7876.302</DistanceMeters><Cadence>81</Cadence><Extensions><TPX xmlns=\"http://www.garmin.com/xmlschemas/ActivityExtension/v2\"><Watts>235</Watts></TPX></Extensions></Trackpoint><Trackpoint><Time>2008-03-03T14:03:07Z</Time><Position><LatitudeDegrees>35.862835</LatitudeDegrees><LongitudeDegrees>-78.902214</LongitudeDegrees></Position><AltitudeMeters>93.385</AltitudeMeters><DistanceMeters>7884.070</DistanceMeters><Cadence>80</Cadence><Extensions><TPX xmlns=\"http://www.garmin.com/xmlschemas/ActivityExtension/v2\"><Watts>230</Watts></TPX></Extensions></Trackpoint><Trackpoint><Time>2008-03-03T14:03:08Z</Time><Position><LatitudeDegrees>35.862858</LatitudeDegrees><LongitudeDegrees>-78.902134</LongitudeDegrees></Position><AltitudeMeters>93.866</AltitudeMeters><DistanceMeters>7891.773</DistanceMeters><Cadence>80</Cadence><Extensions><TPX xmlns=\"http://www.garmin.com/xmlschemas/ActivityExtension/v2\"><Watts>230</Watts></TPX></Extensions></Trackpoint><Trackpoint><Time>2008-03-03T14:03:09Z</Time><Position><LatitudeDegrees>35.862879</LatitudeDegrees><LongitudeDegrees>-78.902054</LongitudeDegrees></Position><AltitudeMeters>93.866</AltitudeMeters><DistanceMeters>7899.320</DistanceMeters><Cadence>79</Cadence><Extensions><TPX xmlns=\"http://www.garmin.com/xmlschemas/ActivityExtension/v2\"><Watts>229</Watts></TPX></Extensions></Trackpoint><Trackpoint><Time>2008-03-03T14:03:10Z</Time><Position><LatitudeDegrees>35.862901</LatitudeDegrees><LongitudeDegrees>-78.901974</LongitudeDegrees></Position><AltitudeMeters>94.347</AltitudeMeters><DistanceMeters>7906.898</DistanceMeters><Cadence>79</Cadence><Extensions><TPX xmlns=\"http://www.garmin.com/xmlschemas/ActivityExtension/v2\"><Watts>228</Watts></TPX></Extensions></Trackpoint><Trackpoint><Time>2008-03-03T14:03:11Z</Time><Position><LatitudeDegrees>35.862928</LatitudeDegrees><LongitudeDegrees>-78.901896</LongitudeDegrees></Position><AltitudeMeters>94.347</AltitudeMeters><DistanceMeters>7914.603</DistanceMeters><Cadence>77</Cadence><Extensions><TPX xmlns=\"http://www.garmin.com/xmlschemas/ActivityExtension/v2\"><Watts>218</Watts></TPX></Extensions></Trackpoint><Trackpoint><Time>2008-03-03T14:03:12Z</Time><Position><LatitudeDegrees>35.862947</LatitudeDegrees><LongitudeDegrees>-78.901817</LongitudeDegrees></Position><AltitudeMeters>94.347</AltitudeMeters><DistanceMeters>7921.995</DistanceMeters><Cadence>77</Cadence><Extensions><TPX xmlns=\"http://www.garmin.com/xmlschemas/ActivityExtension/v2\"><Watts>208</Watts></TPX></Extensions></Trackpoint><Trackpoint><Time>2008-03-03T14:03:13Z</Time><Position><LatitudeDegrees>35.862964</LatitudeDegrees><LongitudeDegrees>-78.901738</LongitudeDegrees></Position><AltitudeMeters>94.347</AltitudeMeters><DistanceMeters>7929.405</DistanceMeters><Cadence>76</Cadence><Extensions><TPX xmlns=\"http://www.garmin.com/xmlschemas/ActivityExtension/v2\"><Watts>190</Wat
